vi "controls_disabled_status.vi"(10 "controls":refnum<vi>[](array[refnum]), 11 "Disabled":T1(ring)) -> ()   [LabVIEW 2016, in "MotionControl.lvlib"]
uses:
  <userlib>/MotionControl/MotionControl.lvlib
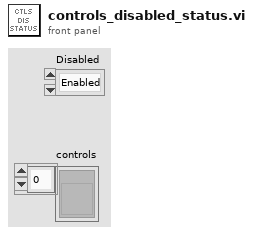
[diagram p1: front panel]
types:
  T1 = enum8{"Enabled", "Disabled", "Disabled and Grayed Out"}
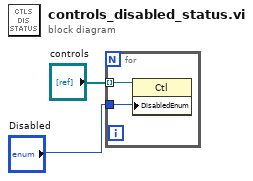
[diagram p0: block diagram]
diagram:
  n1 = for {
    tunnel: "Disabled" -> [w3]
    tunnel: "controls" -> [w4] mode=indexing
    n2 = property class="Ctl"(reference=w4, "DisabledEnum"=w3) -> ()  [unwired: 1 in, 2 out]
  }
